vi "Jogosultságok megnyitás.vi"(8 "error in":errorcluster, 11 "UI Data":T2) -> (0 "error out":errorcluster, 3 "Jogosultsági adatok out":T1[](array[typedef]))   [LabVIEW 2014]
panel:
  out "text":string
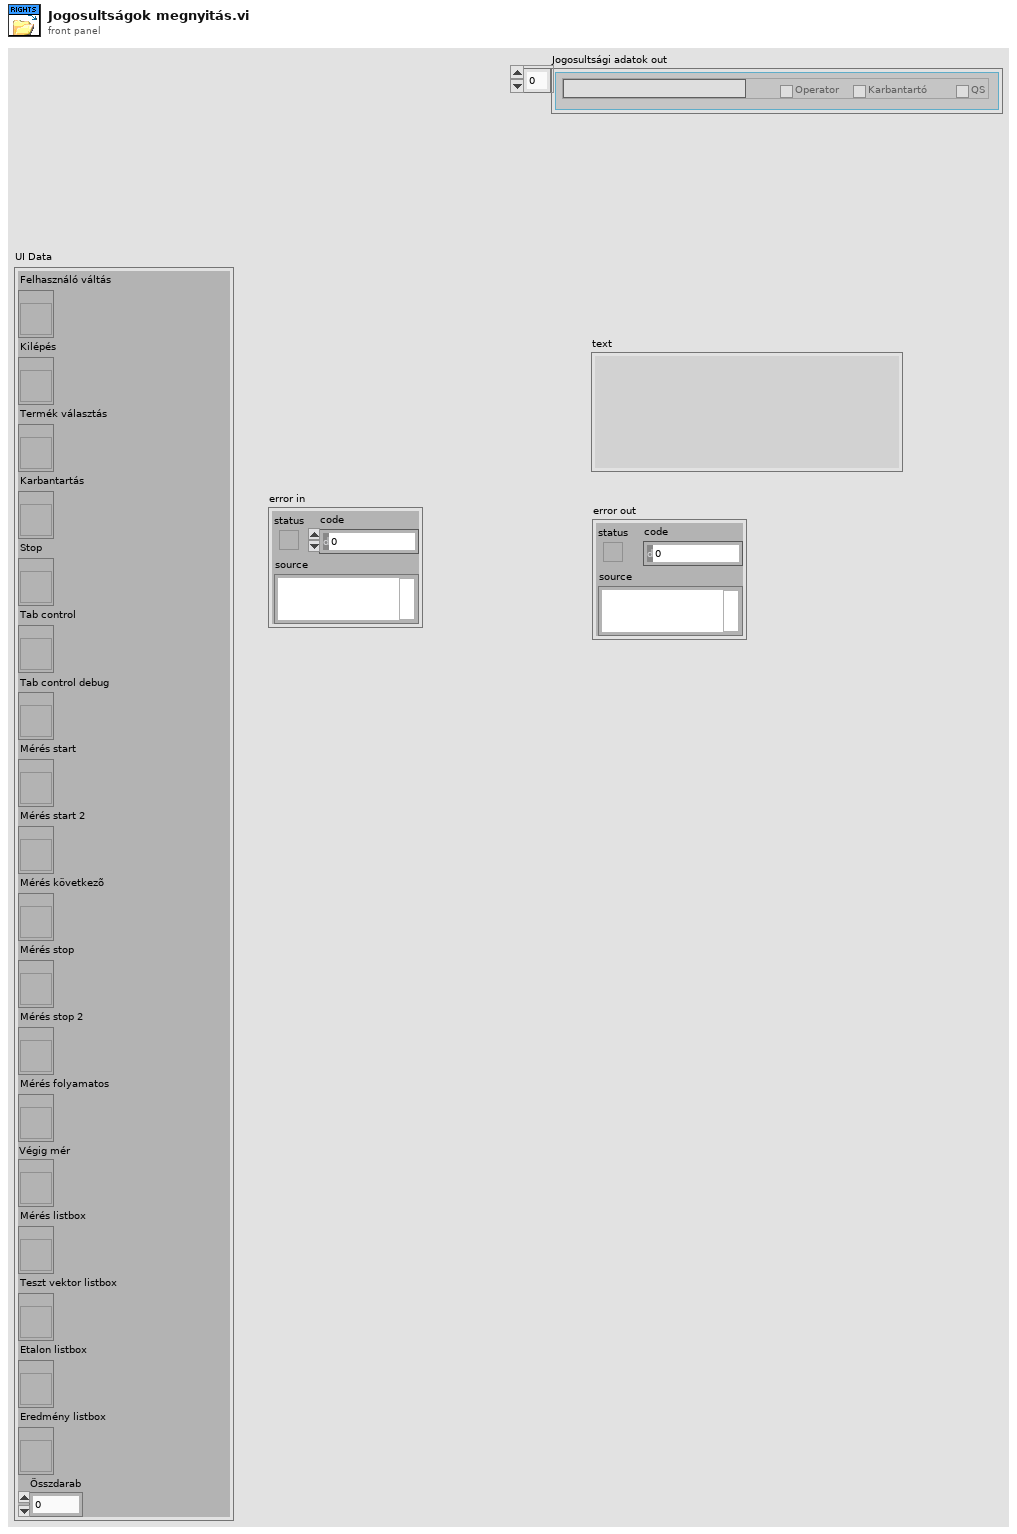
[diagram p1: front panel]
types:
  T1 = typedef "Tab jogosultság.ctl" = cluster{"Tab Name":string, "Operator":bool, "Karbantartó":bool, "QS":bool}
  T2 = typedef "Fõképernyõ references.ctl" = cluster{"Felhasználó váltás":refnum<vi>, "Kilépés":refnum<vi>, "Termék választás":refnum<vi>, "Karbantartás":refnum<vi>, "Stop":refnum<vi>, "Tab control":refnum<vi>, "Tab control debug":refnum<vi>, "Mérés start":refnum<vi>, "Mérés start 2":refnum<vi>, "Mérés következõ":refnum<vi>, "Mérés stop":refnum<vi>, "Mérés stop 2":refnum<vi>, "Mérés folyamatos":refnum<vi>, "Végig mér":refnum<vi>, "Mérés listbox":refnum<vi>, "Teszt vektor listbox":refnum<vi>, "Etalon listbox":refnum<vi>, "Eredmény listbox":refnum<vi>, "Összdarab":i64}
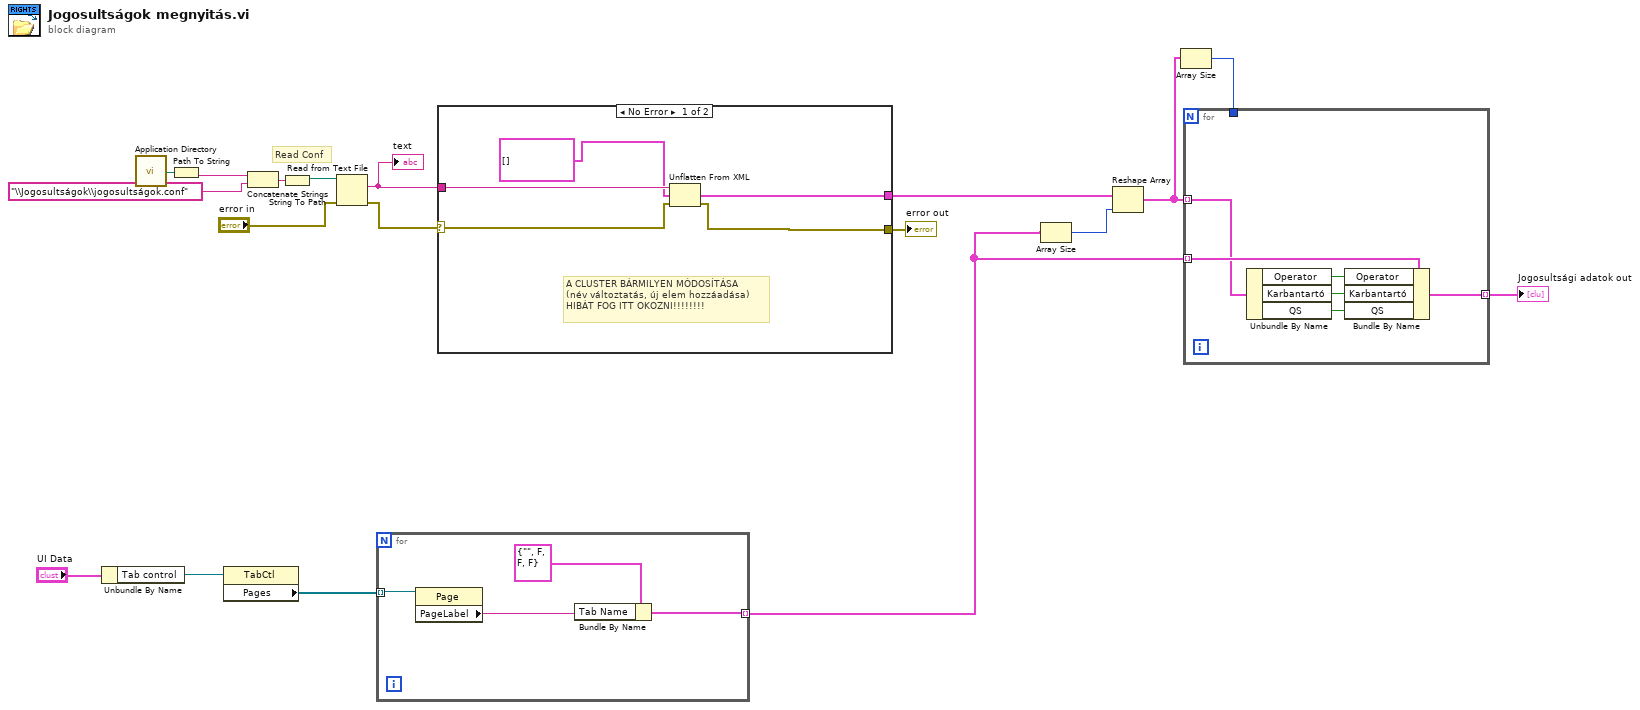
[diagram p0: block diagram]
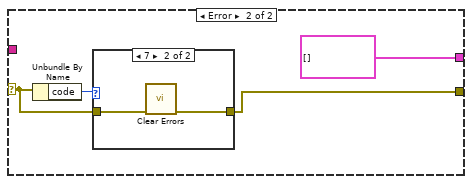
[diagram p2: hidden frame]
diagram:
  # "Read Conf"
  n1 = Unbundle By Name("UI Data") -> ("Tab control"=w17:refnum<vi>)
  n2 = call <vilib>:"Application Directory.vi"() -> ("Application Directory"=w6:path)
  n3 = Path To String(path=w6) -> (string=w4:string)
  n4 = property class="TabCtl"(reference=w17) -> ("Pages"=w16:refnum<vi>[])  [unwired: 1 in, 2 out]
  n5 = Concatenate Strings(w4, "\\Jogosultságok\\jogosultságok.conf" ("prompt (Choose or enter file path)")) -> (w5:string)
  n6 = String To Path(string=w5) -> (path=w2:path)
  n7 = Read from Text File(file (use dialog)=w2, error in="error in") -> (text=w9:string, error out=w1:errorcluster)  [unwired: 2 in, 2 out]
  "text" <- w9
  n8 = for {
    tunnel: w16 -> [w22] mode=indexing
    tunnel: [w19] -> w13 mode=indexing
    n9 = property class="Page"(reference=w22) -> ("PageLabel"=w20:string)  [unwired: 1 in, 2 out]
    n10 = Bundle By Name(cluster=T1 {"Tab Name"="", "Operator"=FALSE, "Karbantartó"=FALSE, "QS"=FALSE} ("Tab engedély"), "Tab Name"=w20) -> (w19:T1)
  }
  n11 = case shown="No Error" w1 {
    selector: w1 -> [w26 w30]
    tunnel: w9 -> [w27 _]
    tunnel: [w25 w29] -> w8
    tunnel: [w23 T1[] []] -> w15
    frame No Error {
      # "A CLUSTER BÁRMILYEN MÓDOSÍTÁSA\n(név változtatás, új elem hozzáadása)\nHIBÁT FOG ITT OKOZNI!!!!!!!!"
      n12 = Unflatten From XML(xml string=w27, type=T1[] [], error in (no error)=w26) -> (value=w23:T1[], error out=w25:errorcluster)
    }
    frame Error {
      n13 = Unbundle By Name(w30) -> ("code"=w31:i32)
      n14 = case shown="7" w31 {
        tunnel: [w32 w33] -> w29
        tunnel: w30 -> [w32 w34]
        frame Default {
        }
        frame 7 {
          n15 = call <vilib>:"Clear Errors.vi"("error in (no error)"=w34) -> ("error out"=w33:errorcluster)  [unwired: 5 in, 1 out]
        }
      }
    }
  }
  "error out" <- w8
  n16 = Array Size(array=w13) -> (size(s)=w14:i32)
  n17 = Reshape Array(w15, w14) -> (w11:T1[])
  n18 = Array Size(array=w11) -> (size(s)=w10:i32)
  n19 = for {
    tunnel: w11 -> [w39] mode=indexing
    tunnel: w13 -> [w40] mode=indexing
    tunnel: [w35] -> w12 mode=indexing
    tunnel: w10 -> [_]
    n20 = Unbundle By Name(w39) -> ("Operator"=w36:bool, "Karbantartó"=w37:bool, "QS"=w38:bool)
    n21 = Bundle By Name(cluster=w40, "Operator"=w36, "Karbantartó"=w37, "QS"=w38) -> (w35:T1)
  }
  "Jogosultsági adatok out" <- w12
